vi "SysLog Viewer aktualisieren.vi"() -> ()   [LabVIEW 2015, in "SysLog.lvlib"]
uses:
  SysLog.lvlib
  Visualisierungs Elemente/Button.ctl
  VI SysLog History.vi
  Allgemein/allgemeine Sub-VIs.lvlib
panel:
  in  "refresh":T1=TRUE caption="quittieren"
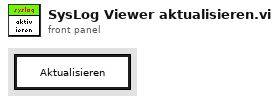
[diagram p1: front panel]
types:
  T1 = typedef "Button.ctl" = bool
  T2 = enum32{"Bad", "Idle", "Run top level", "Running"}
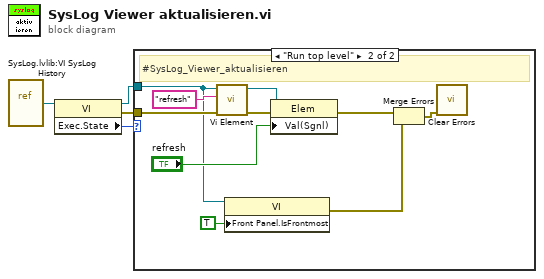
[diagram p0: block diagram]
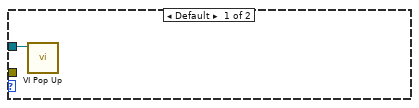
[diagram p2: hidden frame]
diagram:
  n1 = vi-ref "SysLog.lvlib:VI SysLog History.vi"() -> (w2:refnum<vi>)
  n2 = property class="VI"(reference=w2) -> (reference out=w4:refnum<vi>, error out=w3:errorcluster, "Exec.State"=w1:T2)  [unwired: 1 in]
  n3 = case shown="\"Run top level\"" w1 {
    tunnel: w4 -> [w5 w9]
    tunnel: w3 -> [_ w14]
    frame Default {
      n4 = call "VI Pop Up.vi"("VI Referenz"=w5) -> ()  [unwired: 11 in]
    }
    frame "Run top level" {
      # "#SysLog_Viewer_aktualisieren"
      n5 = call "Vi Element.vi"("Fehler (in)"=w14, "Element Beschriftiung"="refresh", "VI Referenz"=w9) -> ("Fehler (out)"=w12:errorcluster, "Elem Referenz"=w13:refnum<vi>)  [unwired: 7 in]
      n6 = property class="VI"(reference=w9, "Front Panel.IsFrontmost"=TRUE ("Frontpanel-Fenster:Ist im Vordergrund")) -> (error out=w6:errorcluster)  [unwired: 1 in, 1 out]
      n7 = property class="Elem"(reference=w13, error in=w12, "Val(Sgnl)"="refresh") -> (error out=w11:errorcluster)  [unwired: 1 out]
      n8 = Merge Errors(w11, w6) -> (w7:errorcluster)
      n9 = call <vilib>:"Clear Errors.vi"("error in (no error)"=w7) -> ()  [unwired: 5 in, 2 out]
    }
  }
